vi "Save exp.vi"(8 "error in (no error)":errorcluster, 10 "save":enum32{"Automatic", "User-def"}(ring), 11 "Control-Client in":refnum<class "Control-Client.lvclass">) -> (0 "error out":errorcluster, 3 "Control-Client out":refnum<class "Control-Client.lvclass">)   [LabVIEW 2015, in "Control-Client.lvclass"]
uses:
  Control-Client.lvclass
  Experiments/Experiment.lvclass/Experiment.ctl
  Control-Client.lvclass/Control-Client.ctl
  Experiments/Experiment.lvclass
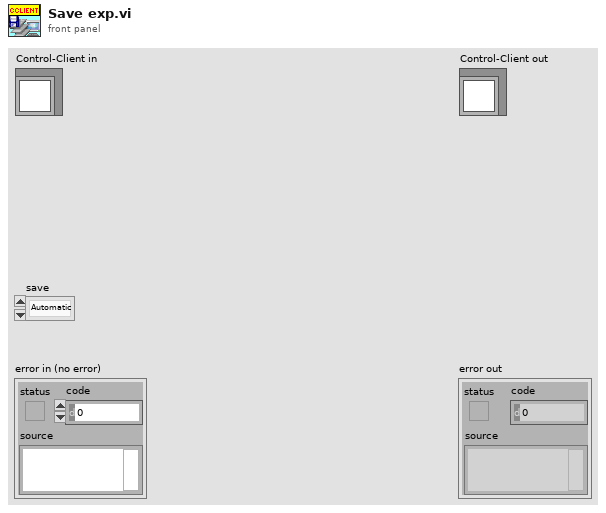
[diagram p1: front panel]
types:
  T1 = enum16{"open", "replace", "create", "open or create", "replace or create", "replace or create with confirmation"}
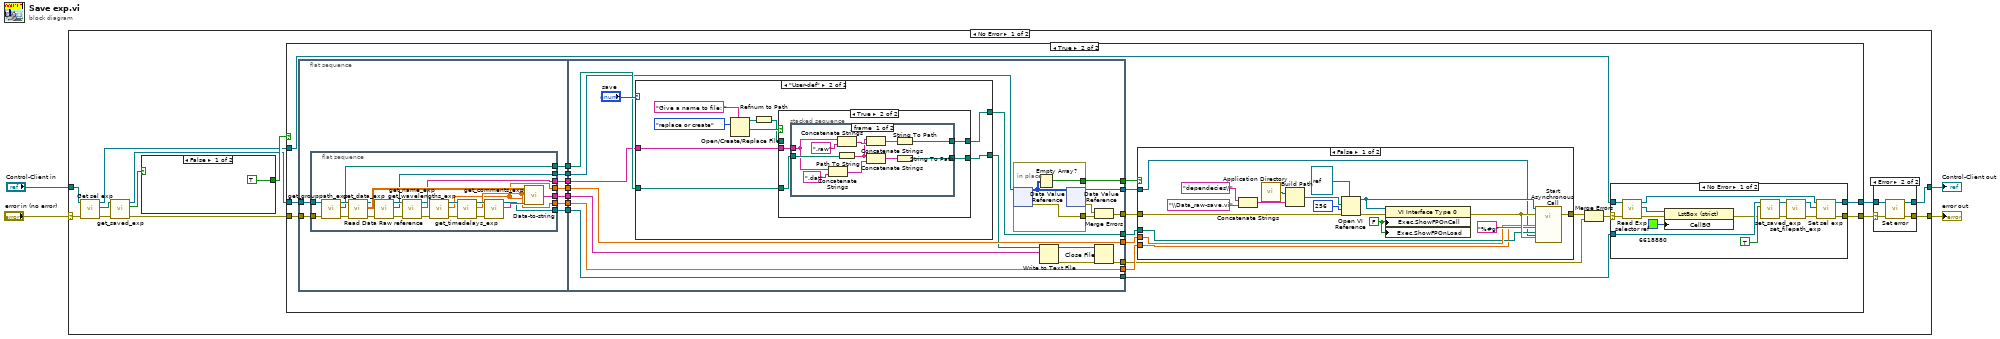
[diagram p0: block diagram]
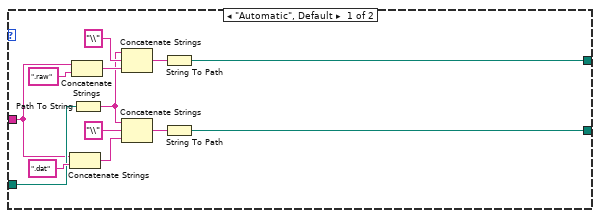
[diagram p4: hidden frame]
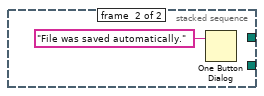
[diagram p6: hidden frame]
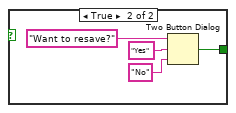
[diagram p9: hidden frame]
diagram:
  n1 = case shown="No Error" "error in (no error)" {
    selector: "error in (no error)" -> [w15 w181]
    tunnel: [w6 w180] -> w2
    tunnel: "Control-Client in" -> [w16 w180]
    tunnel: [w8 w181] -> w1
    frame No Error {
      n2 = call "Get sel exp.vi"("error in (no error)"=w15, "Control-Client in"=w16) -> ("error out"=w13:errorcluster, "Sel experiment"=w14:refnum<class "Experiment.lvclass">, "Control-Client out"=w12:refnum<class "Control-Client.lvclass">)  [unwired: 7 in]
      n3 = call "get_saved_exp.vi"("error in (no error)"=w13, "Experiment.lvclass in"=w14) -> ("error out"=w10:errorcluster, "Saved"=w9:bool, "Experiment.lvclass out"=w11:refnum<class "Experiment.lvclass">)  [unwired: 7 in]
      n4 = case shown="False" w9 {
        tunnel: [TRUE ("T button?") w176] -> w17
        frame False {
        }
        frame True {
          n5 = Two Button Dialog(message="Want to resave?", 1:"No" ("F button name (\"Cancel\")"), 2:"Yes" ("T button name (\"OK\")")) -> (T button?=w176:bool)
        }
      }
      n6 = case shown="True" w17 {
        tunnel: w11 -> [_ w42]
        tunnel: w10 -> [w25 w47]
        tunnel: [w25 w44] -> w5
        tunnel: [w24 w43] -> w7
        tunnel: w12 -> [w24 w46]
        frame False {
        }
        frame True {
          n7 = flat-sequence {
            tunnel: w47 -> [w55]
            tunnel: w42 -> [w51]
            tunnel: [w56] -> w37
            tunnel: [w54] -> w36
            tunnel: [w53] -> w35
            tunnel: [w52] -> w34
            tunnel: [w50] -> w33
            tunnel: [w49] -> w32
            tunnel: [w48] -> w31
            tunnel: [w95] -> w40
            tunnel: [w96] -> w41
            tunnel: [w97] -> w45
            tunnel: w37 -> [w87]
            tunnel: w36 -> [w93]
            tunnel: w35 -> [w92]
            tunnel: w34 -> [w97]
            tunnel: w33 -> [w96]
            tunnel: w32 -> [w95]
            tunnel: w31 -> [w84]
            tunnel: [w91] -> w30
            tunnel: [w86] -> w29
            tunnel: [w85] -> w28
            tunnel: [w81] -> w27
            tunnel: [w80] -> w26
            frame #0 {
              n8 = flat-sequence {
                tunnel: [w73] -> w56
                tunnel: w55 -> [w71]
                tunnel: [w68] -> w54
                tunnel: [w67] -> w53
                tunnel: [w65] -> w52
                tunnel: w51 -> [w64]
                tunnel: [w63] -> w50
                tunnel: [w62] -> w49
                tunnel: [w57] -> w48
                frame #0 {
                  n9 = call "get_grouppath_exp.vi"("error in (no error)"=w71, "Experiment.lvclass in"=w64) -> ("error out"=w70:errorcluster, "GroupPath"=w68:path, "Experiment.lvclass out"=w69:refnum<class "Experiment.lvclass">)  [unwired: 7 in]
                  n10 = call "get_data_exp.vi"("error in (no error)"=w70, "Experiment.lvclass in"=w69) -> ("error out"=w61:errorcluster, "Data"=w75:sgl[][], "Experiment.lvclass out"=w58:refnum<class "Experiment.lvclass">)  [unwired: 7 in]
                  n11 = call "Read Data Raw reference.vi"("error in (no error)"=w61, "Experiment in"=w58) -> ("error out"=w60:errorcluster, "Data Raw reference"=w57:refnum<data-value>, "Experiment out"=w59:refnum<class "Experiment.lvclass">)  [unwired: 7 in]
                  n12 = call "get_name_exp.vi"("error in (no error)"=w60, "Experiment.lvclass in"=w59) -> ("error out"=w72:errorcluster, "Exp name"=w67:string, "Experiment.lvclass out"=w66:refnum<class "Experiment.lvclass">)  [unwired: 7 in]
                  n13 = call "get_wavelengths_exp.vi"("error in (no error)"=w72, "Experiment.lvclass in"=w66) -> ("error out"=w77:errorcluster, "wavelengths"=w62:dbl[], "Experiment.lvclass out"=w76:refnum<class "Experiment.lvclass">)  [unwired: 7 in]
                  n14 = call "get_timedelays_exp.vi"("error in (no error)"=w77, "Experiment.lvclass in"=w76) -> ("error out"=w78:errorcluster, "timedelays"=w63:dbl[], "Experiment.lvclass out"=w79:refnum<class "Experiment.lvclass">)  [unwired: 7 in]
                  n15 = call "get_comments_exp.vi"("error in (no error)"=w78, "Experiment.lvclass in"=w79) -> ("Comments"=w74:string, "Experiment.lvclass out"=w65:refnum<class "Experiment.lvclass">)  [unwired: 7 in, 1 out]
                  n16 = call "Data-to-string.vi"("Comments"=w74, "wavelength"=w62, "timedelay"=w63, "DATA"=w75) -> ("resulted string"=w73:string)
                }
              }
            }
            frame #1 {
              n17 = case shown="\"User-def\"" "save" {
                tunnel: w93 -> [w104 w116]
                tunnel: [w111 w118] -> w88
                tunnel: w92 -> [w103 w115]
                tunnel: [w102 w114] -> w91
                frame "Automatic", Default {
                  n18 = Concatenate Strings(w103, ".dat" ("string")) -> (w110:string)
                  n19 = Concatenate Strings(w103, ".raw" ("string")) -> (w107:string)
                  n20 = Path To String(path=w104) -> (string=w101:string)
                  n21 = Concatenate Strings(w101, "\\" ("string"), w107) -> (w106:string)
                  n22 = Concatenate Strings(w101, "\\" ("string"), w110) -> (w112:string)
                  n23 = String To Path(string=w106) -> (path=w102:path)
                  n24 = String To Path(string=w112) -> (path=w111:path)
                }
                frame "User-def" {
                  n25 = Open/Create/Replace File(prompt="Give a name to file: ", operation (0:open)=T1."replace or create") -> (refnum out=w120:refnum<file>, cancelled=w119:bool)  [unwired: 4 in, 1 out]
                  n26 = Refnum to Path(1:w120) -> (0:w117:path)
                  n27 = case shown="True" w119 {
                    tunnel: [w123 w127] -> w118
                    tunnel: w117 -> [w123 _]
                    tunnel: w116 -> [_ w126]
                    tunnel: w115 -> [_ w125]
                    tunnel: [w123 w124] -> w114
                    frame False {
                    }
                    frame True {
                      n28 = stacked-sequence {
                        tunnel: [w135 _] -> w127
                        tunnel: w126 -> [w134 _]
                        tunnel: w125 -> [w129 _]
                        tunnel: [w128 _] -> w124
                        frame #0 {
                          n29 = Concatenate Strings(w129, ".dat" ("string")) -> (w137:string)
                          n30 = Concatenate Strings(w129, ".raw" ("string")) -> (w132:string)
                          n31 = Path To String(path=w134) -> (string=w130:string)
                          n32 = Concatenate Strings(w130, w132) -> (w133:string)
                          n33 = Concatenate Strings(w130, w137) -> (w136:string)
                          n34 = String To Path(string=w133) -> (path=w128:path)
                          n35 = String To Path(string=w136) -> (path=w135:path)
                        }
                        frame #1 {
                          n36 = One Button Dialog(message="File was saved automatically.") -> ()  [unwired: 1 in, 1 out]
                        }
                      }
                    }
                  }
                }
              }
              n37 = in-place {
                in-place-border: [w100] -> w80
                in-place-border: [w99] -> w83
                n38 = in-place-dvr #1(w84) -> (w98:i32[][][][], w99:errorcluster)
                n39 = Empty Array?(array=w98) -> (empty?=w100:bool)
                n40 = in-place-dvr #1(w98) -> (w85:refnum<data-value>, w82:errorcluster)
              }
              n41 = Write to Text File(file (use dialog)=w88, text=w87) -> (refnum out=w89:refnum<file>, error out=w90:errorcluster)  [unwired: 2 in, 1 out]
              n42 = Merge Errors(w82, w83) -> (w81:errorcluster)
              n43 = Close File(refnum=w89, error in=w90) -> (error out=w86:errorcluster)  [unwired: 1 out]
            }
          }
          n44 = case shown="False" w26 {
            tunnel: w40 -> [w145 _]
            tunnel: w30 -> [w144 _]
            tunnel: [w143 _] -> w38
            tunnel: w41 -> [w142 _]
            tunnel: w27 -> [w141 _]
            tunnel: w28 -> [w140 _]
            frame False {
              w153 = FALSE ("Execution:Show Front Panel On Call")
              n45 = Concatenate Strings("dependecies\\" ("chaîne"), "\\Data_raw-save.vi" ("chaîne")) -> (w149:string)
              n46 = call <vilib>:"Application Directory.vi"() -> ("Application Directory"=w150:path)
              n47 = Build Path(base path=w150, name or relative path=w149) -> (appended path=w146:path)
              n48 = Open VI Reference(type specifier VI Refnum (for type only)=refnum<vi> refnum ("spécificateur de type du refnum de VI (pour type seulement)"), vi path=w146, options=256, error in (no error)=w141) -> (vi reference=w154:refnum<vi>, error out=w152:errorcluster)  [unwired: 2 in]
              n49 = property class="VI Interface Type 0"(reference=w154, error in=w152, "Exec.ShowFPOnCall"=w153, "Exec.ShowFPOnLoad"=w153) -> (error out=w156:errorcluster)  [unwired: 1 out]
              n50 = call-by-ref "Start Asynchronous Call"(reference=w154, error in=w156, "timedelay"=w142, "data value reference"=w140, "wavelength"=w145, "error in"=w156, "file (use dialog)"=w144, "accuracy"="%#g") -> (error out=w143:errorcluster)  [unwired: 5 in, 2 out]
            }
            frame True {
            }
          }
          n51 = Merge Errors(w38, w29) -> (w39:errorcluster)
          n52 = case shown="No Error" w39 {
            selector: w39 -> [w171 w174]
            tunnel: [w158 w174] -> w44
            tunnel: w46 -> [w169 w173]
            tunnel: w45 -> [w172 _]
            tunnel: [w170 w173] -> w43
            frame No Error {
              n53 = call "Read Exp selector ref.vi"("error in (no error)"=w171, "Control-Client in"=w169) -> ("error out"=w164:errorcluster, "Exp selector ref"=w168:refnum<vi>, "Control-Client out"=w162:refnum<class "Control-Client.lvclass">)  [unwired: 7 in]
              n54 = property class="LstBox (strict)"(reference=w168, error in=w164, "CellBG"=u32 6618880) -> (error out=w159:errorcluster)  [unwired: 1 out]
              n55 = call "set_saved_exp.vi"("error in (no error)"=w159, "Saved"=TRUE, "Experiment.lvclass in"=w172) -> ("error out"=w166:errorcluster, "Experiment.lvclass out"=w165:refnum<class "Experiment.lvclass">)  [unwired: 7 in]
              n56 = call "set_filepath_exp.vi"("error in (no error)"=w166, "Experiment.lvclass in"=w165) -> ("error out"=w160:errorcluster, "Experiment.lvclass out"=w161:refnum<class "Experiment.lvclass">)  [unwired: 8 in]
              n57 = call "Set sel exp.vi"("error in (no error)"=w160, "Experiment"=w161, "Control-Client in"=w162) -> ("error out"=w158:errorcluster, "Control-Client out"=w170:refnum<class "Control-Client.lvclass">)  [unwired: 7 in]
            }
            frame Error {
            }
          }
        }
      }
      n58 = case shown="Error" w5 {
        selector: w5 -> [w19 w20]
        tunnel: [w19 w23] -> w8
        tunnel: w7 -> [w18 w22]
        tunnel: [w18 w21] -> w6
        frame No Error {
        }
        frame Error {
          n59 = call "Set error.vi"("error in (no error)"=w20, "Control-Client in"=w22) -> ("error out"=w23:errorcluster, "Control-Client out"=w21:refnum<class "Control-Client.lvclass">)  [unwired: 8 in]
        }
      }
    }
    frame Error {
    }
  }
  "error out" <- w1
  "Control-Client out" <- w2
